vi "Recalibration.vi"() -> ()   [LabVIEW 2012]
uses:
  <vilib>/Utility/file.llb/Read From Spreadsheet File (I64).vi
  <vilib>/Utility/file.llb/Write To Spreadsheet File (DBL).vi
panel:
  in  "stop":bool
  in  "New\nCalibration #":i32=1 min=1 max=100 step=1
  in  "Correct and Save":bool
  in  "Apply Calibration":bool
  out "Calibration Does Not Exist":bool
  in  "Load Button":bool
  out "Suggested Cal #":i32
  in  "Tolerance (°)":dbl=30.0 min=0.0
  out "Bad Min":bool[](array[boolean])
  out "Bad Max":bool[](array[boolean])
  in  "Calibration #":i32=1 min=1 max=100 step=1
  out "Min Deg":dbl[](array[numeric])
  out "Max Deg":dbl[](array[numeric])
  out "Joint Name":string[](array[string])=["Thumb Roll", "Thumb Inner", "Thumb Outer", "Thm-Ind Abd", "Index MCP", "Index PIP", "Middle MCP", "Middle PIP", "Ind-Mid Abd", "Ring MCP", "Ring PIP", "Mid-Rng Abd", "Pinkie MCP", "Pinkie PIP", "Rng-Pnk Abduction", "Wrist Pitch", "Wrist Yaw"]
  out "Min Raw":i64[](array[numeric])
  out "Max Raw":i64[](array[numeric])
  in  "Hand":string(combo)="LH"
  in  "Subject Initials":string="Default"
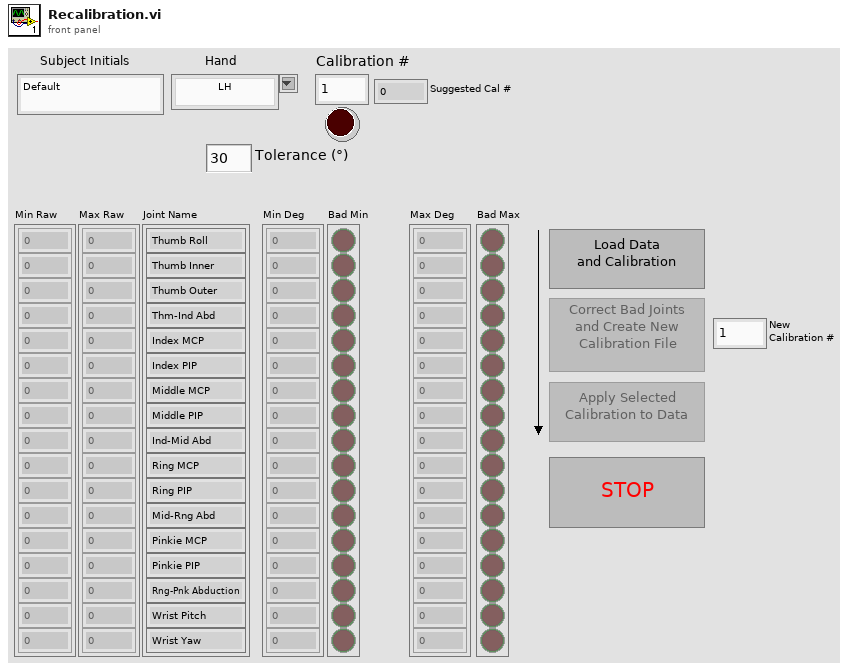
[diagram p1: front panel]
types:
  T1 = enum8{"Enabled", "Disabled", "Disabled and Grayed Out"}
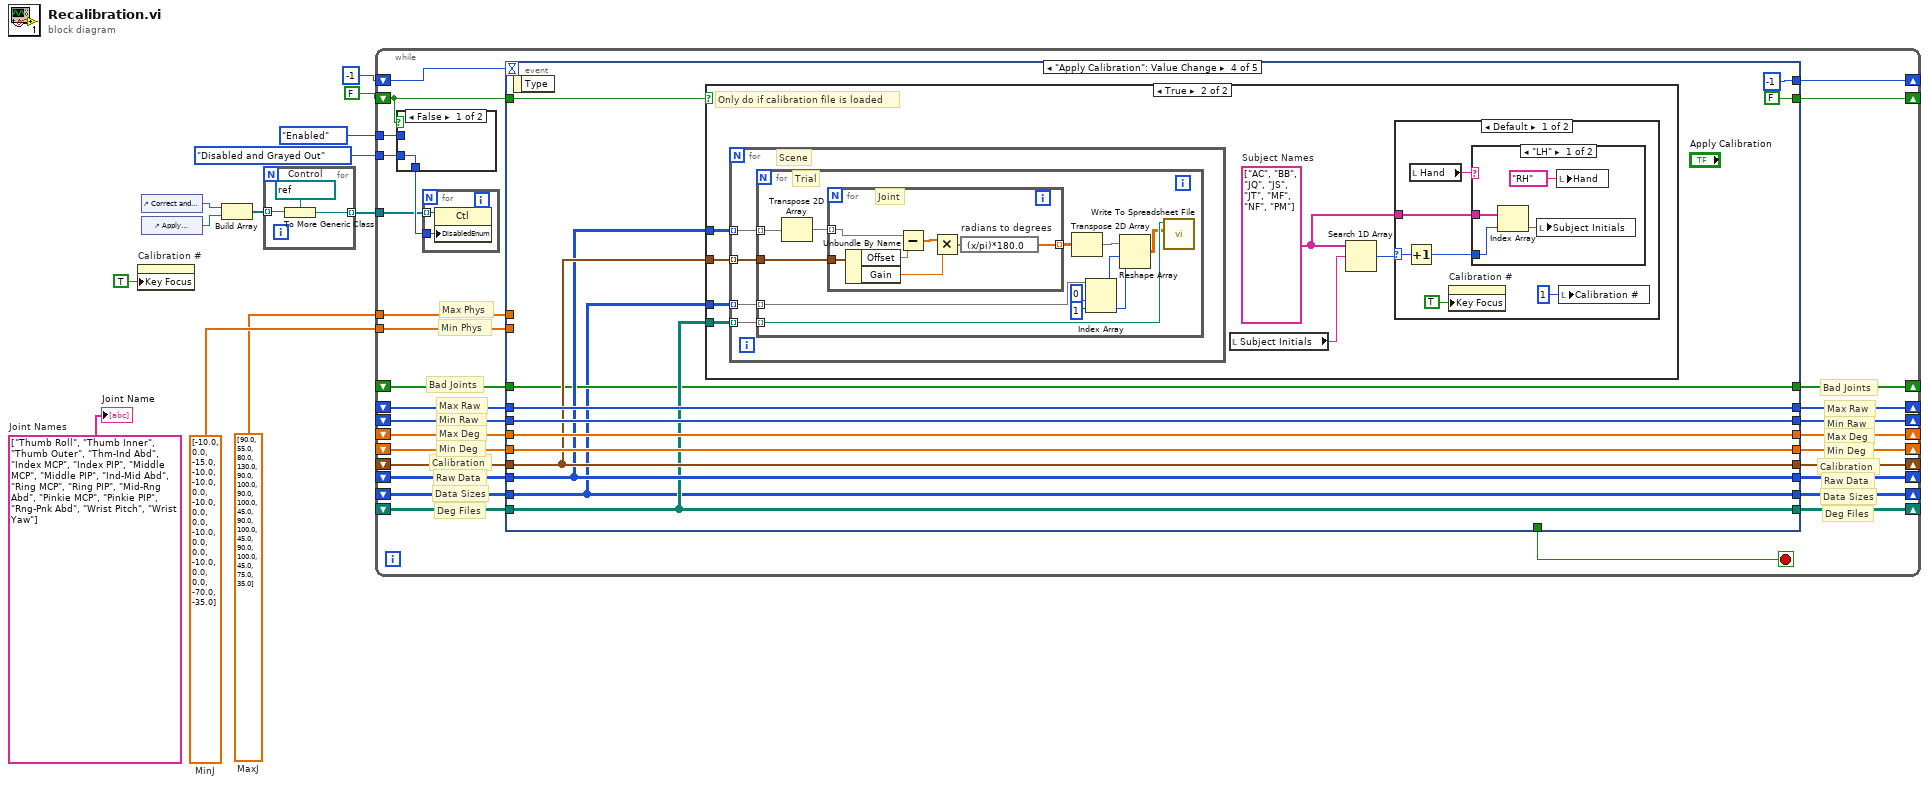
[diagram p0: block diagram]
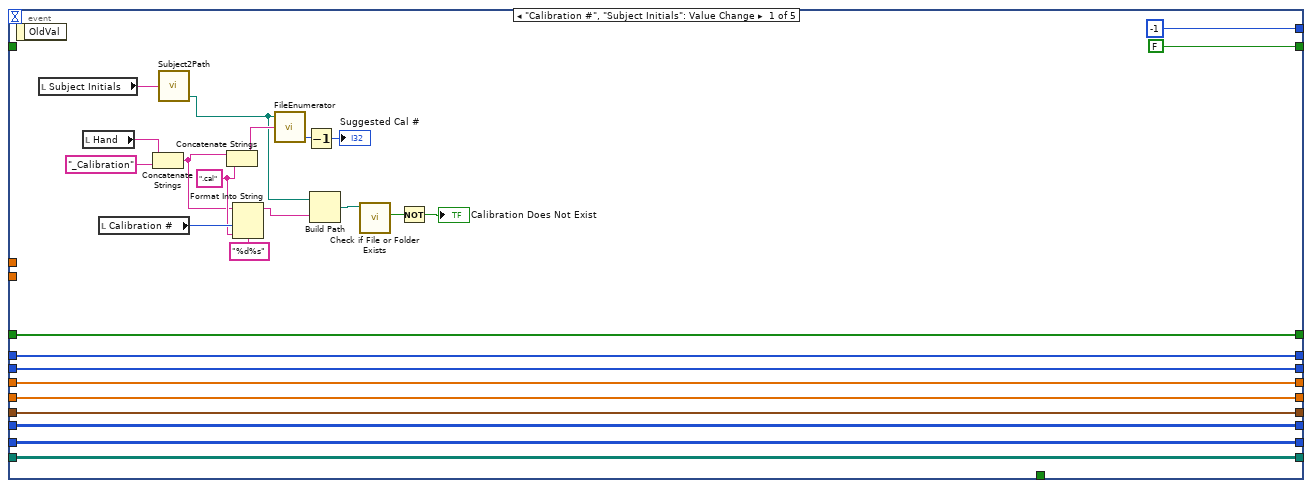
[diagram p3: hidden frame]
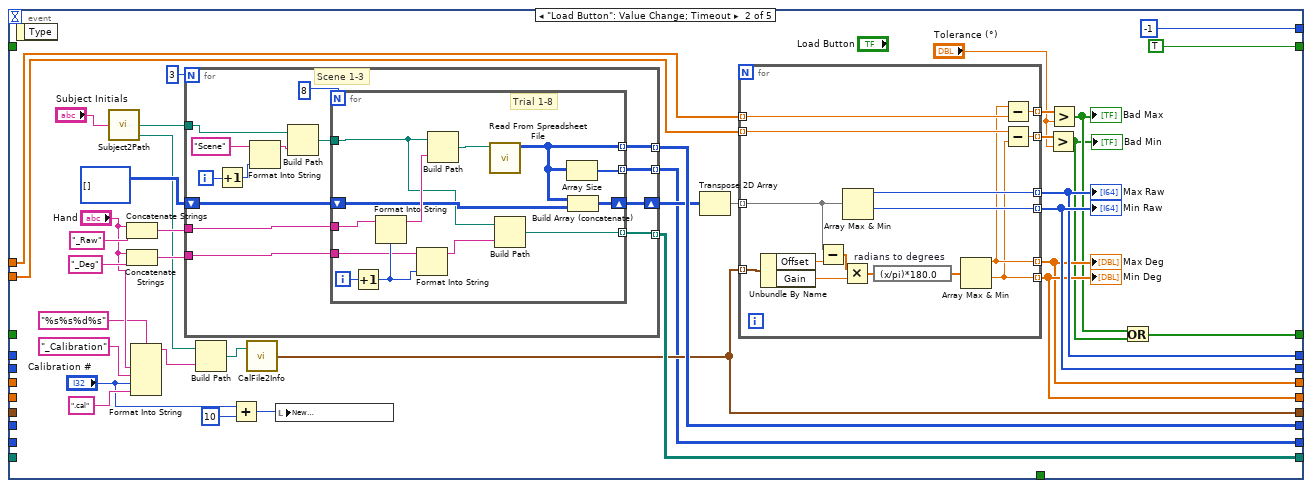
[diagram p4: hidden frame]
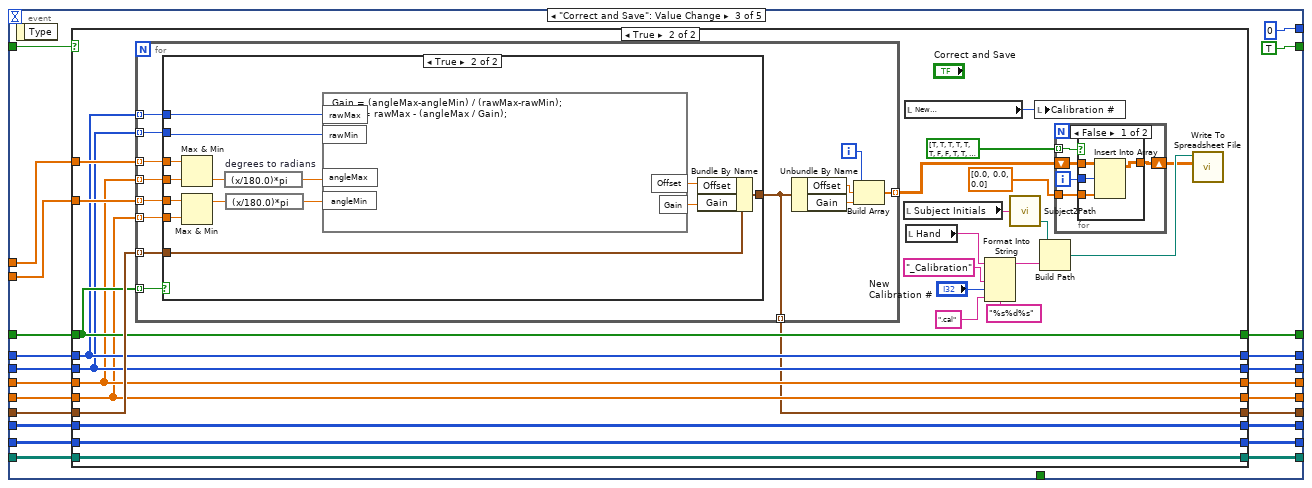
[diagram p5: hidden frame]
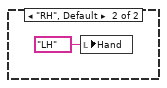
[diagram p10: hidden frame]
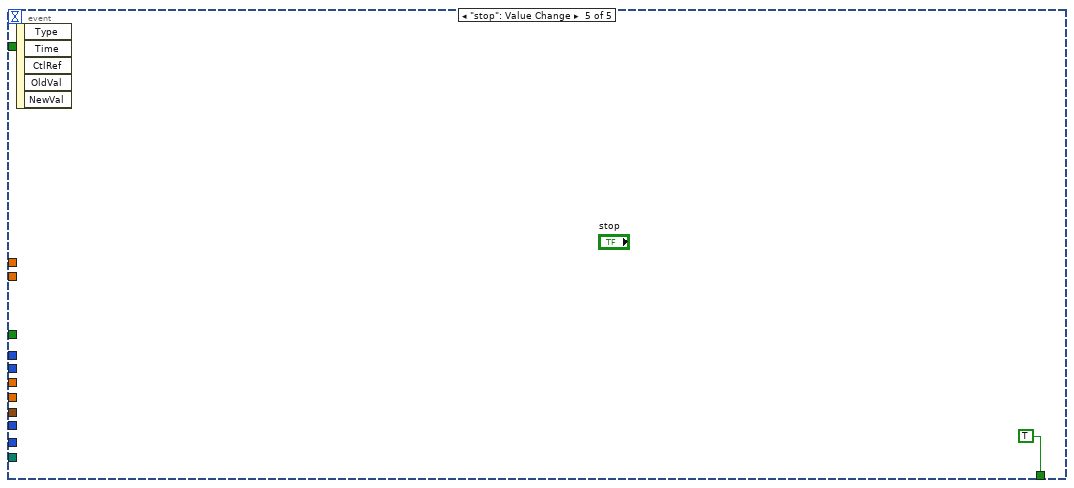
[diagram p12: hidden frame]
diagram:
  w9 = dbl[] [90.0, 55.0, 80.0, 130.0, 90.0, 100.0, 90.0, 100.0, 45.0, 90.0, 100.0, 45.0, 90.0, 100.0, 45.0, 75.0, 35.0]  # MaxJ
  w10 = dbl[] [-10.0, 0.0, -15.0, -10.0, -10.0, 0.0, -10.0, 0.0, 0.0, -10.0, 0.0, 0.0, -10.0, 0.0, 0.0, -70.0, -35.0]  # MinJ
  w11 = string[] ["Thumb Roll", "Thumb Inner", "Thumb Outer", "Thm-Ind Abd", "Index MCP", "Index PIP", "Middle MCP", "Middle PIP", "Ind-Mid Abd", "Ring MCP", "Ring PIP", "Mid-Rng Abd", "Pinkie MCP", "Pinkie PIP", "Rng-Pnk Abd", "Wrist Pitch", "Wrist Yaw"]  # Joint Names
  n1 = property on="Calibration #" class="DigNum (strict)"("Key Focus"=TRUE) -> ()  [unwired: 2 in, 2 out]
  n2 = control-ref of="Correct and Save"() -> (w7:refnum<vi>)
  n3 = control-ref of="Apply Calibration"() -> (w6:refnum<vi>)
  n4 = Build Array(w7, w6) -> (w5:refnum<vi>[])
  n5 = for {
    tunnel: w5 -> [w15] mode=indexing
    tunnel: [w13] -> w2 mode=indexing
    w14 = refnum<vi> refnum  # Control
    n6 = To More Generic Class(target class=w14, reference=w15) -> (generic class reference=w13:refnum<vi>)
  }
  n7 = while {
    shift-right: [w44] -> _
    shift-left: _ -> [w43]
    shift-right: [w42] -> _
    shift-left: _ -> [w31]
    shift-right: [w41] -> _
    shift-left: _ -> [w32]
    shift-right: [w37] -> _
    shift-left: _ -> [w33]
    shift-right: [w38] -> _
    shift-left: _ -> [w34]
    shift-right: [w39] -> _
    shift-left: _ -> [w35]
    shift-right: [w40] -> _
    shift-left: _ -> [w36]
    shift-right: [w30] -> _
    shift-left: FALSE ("Load Button") -> [w20]
    tunnel: w10 -> [w29]
    tunnel: w9 -> [w28]
    shift-right: [w27] -> _
    shift-left: _ -> [w26]
    shift-right: [w25] -> _
    shift-left: -1 -> [w24]
    shift-right: [w22] -> _
    shift-left: _ -> [w21]
    tunnel: T1."Enabled" ("Disabled") -> [w19]
    tunnel: T1."Disabled and Grayed Out" ("Disabled") -> [w18]
    tunnel: w2 -> [w16]
    stop <- w23 stop-if-true
    # "Data Sizes"
    # "Data Sizes"
    # "Bad Joints"
    # "Bad Joints"
    # "Min Phys"
    # "Max Phys"
    # "Deg Files"
    # "Raw Data"
    # "Calibration"
    # "Min Deg"
    # "Max Deg"
    # "Min Raw"
    # "Max Raw"
    # "Deg Files"
    # "Raw Data"
    # "Calibration"
    # "Min Deg"
    # "Max Deg"
    # "Min Raw"
    # "Max Raw"
    n8 = case shown="False" w20 {
      tunnel: w19 -> [_ w48]
      tunnel: w18 -> [w47 _]
      tunnel: [w47 w48] -> w17
      frame False {
      }
      frame True {
      }
    }
    n9 = for {
      tunnel: w17 -> [w46]
      tunnel: w16 -> [w45] mode=indexing
      n10 = property class="Ctl"(reference=w45, "DisabledEnum"=w46) -> ()  [unwired: 1 in, 2 out]
    }
    n11 = event shown="[3] \"Apply Calibration\": Value Change" {
      selector: _ -> [_ _ _ _ _]
      dyn-events: _ -> [_ _ _ _ _]
      timeout: w24 -> [_ _ _ _ _]
      tunnel: [w69 w95 w166 w258 _] -> w44
      tunnel: w43 -> [w69 _ w171 w258 _]
      tunnel: [w63 w98 w169 w256 _] -> w42
      tunnel: [w64 w97 w167 w257 _] -> w41
      tunnel: [w68 w92 w162 w262 _] -> w40
      tunnel: [w67 w93 w163 w261 _] -> w39
      tunnel: [w66 w90 w164 w260 _] -> w38
      tunnel: [w65 w91 w165 w259 _] -> w37
      tunnel: w36 -> [w68 _ w175 w262 _]
      tunnel: w35 -> [w67 _ w174 w261 _]
      tunnel: w34 -> [w66 _ w173 w260 _]
      tunnel: w33 -> [w65 _ w172 w259 _]
      tunnel: w32 -> [w64 _ w170 w257 _]
      tunnel: w31 -> [w63 _ w168 w256 _]
      tunnel: [FALSE ("Load Button") TRUE ("Load Button") TRUE ("Load Button") FALSE ("Load Button") _] -> w30
      tunnel: w20 -> [_ _ w177 w255 _]
      tunnel: w29 -> [_ w87 w159 _ _]
      tunnel: w28 -> [_ w88 w160 _ _]
      tunnel: [w52 w78 w161 w254 _] -> w27
      tunnel: w26 -> [w52 _ w176 w254 _]
      tunnel: [-1 -1 0 -1 _] -> w25
      tunnel: [_ _ _ _ TRUE] -> w23
      tunnel: [w49 w75 w155 w251 _] -> w22
      tunnel: w21 -> [w49 _ w156 w251 _]
      event "Calibration #", "Subject Initials": Value Change {
        w60 = ".cal"
        n12 = event-data() -> ()  [unwired: 1 in, 1 out]
        n13 = local read "Subject Initials"() -> (w74:string)
        n14 = local read "Hand"() -> (w73:string)
        n15 = local read "Calibration #"() -> (w61:i32)
        n16 = Concatenate Strings(w73, "_Calibration") -> (w59:string)
        n17 = call "Subject2Path.vi"("Subject Initials"=w74) -> ("Calibration Path"=w57:path)  [unwired: 1 in, 2 out]
        n18 = Concatenate Strings(w59, w60) -> (w62:string)
        n19 = Format Into String(format string="%d%s", initial string=w59, w61, w60) -> (resulting string=w56:string)  [unwired: 1 in, 1 out]
        n20 = call "FileEnumerator.vi"("Filename"=w62, "Path"=w57) -> ("Number"=w70:i32)  [unwired: 1 in, 2 out]
        n21 = Decrement(x=w70) -> (x-1=→"Suggested Cal #":i32)
        n22 = Build Path(base path=w57, name or relative path=w56) -> (appended path=w55:path)
        n23 = call <vilib>:"Check if File or Folder Exists.vi"("path"=w55) -> ("file or folder exists?"=w54:bool)  [unwired: 8 in, 2 out]
        n24 = Not(x=w54) -> (.not. x?=→"Calibration Does Not Exist":bool)
      }
      event "Load Button": Value Change; Timeout {
        n25 = event-data() -> ()  [unwired: 1 in, 1 out]
        n26 = call "Subject2Path.vi"("Subject Initials"="Subject Initials") -> ("Data Path"=w105:path, "Calibration Path"=w100:path)  [unwired: 1 in, 1 out]
        n27 = Concatenate Strings("Hand", "_Raw") -> (w108:string)
        n28 = Concatenate Strings("Hand", "_Deg") -> (w107:string)
        n29 = Format Into String(format string="%s%s%d%s", "Hand", "_Calibration", "Calibration #", ".cal") -> (resulting string=w99:string)  [unwired: 2 in, 1 out]
        n30 = for {
          N: 3 -> [_]
          tunnel: w105 -> [w138]
          tunnel: w108 -> [w136]
          shift-right: [w132] -> w96
          shift-left: i64[][] [] ("array") -> [w133]
          tunnel: [w131] -> w97 mode=indexing
          tunnel: w107 -> [w130]
          tunnel: [w129] -> w98 mode=indexing
          tunnel: [w128] -> w75 mode=indexing
          i -> [w140]
          # "Scene 1-3"
          n31 = Increment(x=w140) -> (x+1=w139:i32)
          n32 = Format Into String(initial string="Scene", w139) -> (resulting string=w134:string)  [unwired: 2 in, 1 out]
          n33 = Build Path(base path=w138, name or relative path=w134) -> (appended path=w137:path)
          n34 = for {
            N: 8 -> [_]
            tunnel: w137 -> [w146]
            tunnel: w136 -> [w153]
            shift-right: [w149] -> w132
            shift-left: w133 -> [w150]
            tunnel: [w143] -> w131 mode=indexing
            tunnel: w130 -> [w147]
            tunnel: [w144] -> w129 mode=indexing
            tunnel: [w142] -> w128 mode=indexing
            i -> [w154]
            # "Trial 1-8"
            n35 = Increment(x=w154) -> (x+1=w148:i32)
            n36 = Format Into String(initial string=w153, w148) -> (resulting string=w152:string)  [unwired: 2 in, 1 out]
            n37 = Format Into String(initial string=w147, w148) -> (resulting string=w145:string)  [unwired: 2 in, 1 out]
            n38 = Build Path(base path=w146, name or relative path=w152) -> (appended path=w151:path)
            n39 = call-poly <vilib>:"Read From Spreadsheet File.vi"("file path (dialog if empty)"=w151) -> ("all rows"=w143:i64[][])  [unwired: 6 in, 4 out]
            n40 = Build Path(base path=w146, name or relative path=w145) -> (appended path=w144:path)
            n41 = Array Size(array=w143) -> (size(s)=w142:i32[])
            n42 = Build Array (concatenate)(w143, w150) -> (w149:i64[][])
          }
        }
        n43 = Build Path(base path=w100, name or relative path=w99) -> (appended path=w89:path)
        n44 = Add(x="Calibration #", y=10) -> (x+y=w81:i32)
        n45 = call "CalFile2Info.vi"("Calibration File"=w89) -> ("Calibration Array"=w95:cluster{"Offset":dbl, "Gain":dbl}[])  [unwired: 3 in]
        n46 = local write "New\nCalibration #"(w81) -> ()
        n47 = Transpose 2D Array(2D array=w96) -> (transposed array=w94:i64[][])
        n48 = for {
          tunnel: w95 -> [w127] mode=indexing
          tunnel: w94 -> [w121] mode=indexing
          tunnel: [w120] -> w92 mode=indexing
          tunnel: [w119] -> w93 mode=indexing
          tunnel: [w116] -> w90 mode=indexing
          tunnel: [w115] -> w91 mode=indexing
          tunnel: w88 -> [w118] mode=indexing
          tunnel: w87 -> [w117] mode=indexing
          tunnel: [w114] -> w86 mode=indexing
          tunnel: [w113] -> w85 mode=indexing
          n49 = Unbundle By Name(w127) -> ("Offset"=w126:dbl, "Gain"=w125:dbl)
          n50 = Subtract(x=w121, y=w126) -> (x-y=w124:dbl[])
          n51 = Multiply(x=w124, y=w125) -> (x*y=w123:dbl[])
          n52 = Array Max & Min(array=w121) -> (max value=w120:i64, min value=w119:i64)  [unwired: 2 out]
          n53 = expression code="(x/pi)*180.0" "radians to degrees"(w123) -> (w122:dbl[])
          n54 = Array Max & Min(array=w122) -> (max value=w116:dbl, min value=w115:dbl)  [unwired: 2 out]
          n55 = Subtract(x=w116, y=w118) -> (x-y=w114:dbl)
          n56 = Subtract(x=w117, y=w115) -> (x-y=w113:dbl)
        }
        "Min Raw" <- w93
        "Max Raw" <- w92
        "Min Deg" <- w91
        "Max Deg" <- w90
        n57 = Greater?(x=w85, y="Tolerance (°)") -> (0:w79:bool[])
        "Bad Min" <- w79
        n58 = Greater?(x=w86, y="Tolerance (°)") -> (0:w80:bool[])
        "Bad Max" <- w80
        n59 = Or(x=w80, y=w79) -> (x .or. y?=w78:bool[])
      }
      event "Correct and Save": Value Change {
        n60 = event-data() -> ()  [unwired: 1 in, 1 out]
        n61 = case shown="True" w177 {
          tunnel: [w186 w207] -> w161
          tunnel: w176 -> [w186 w207]
          tunnel: [w185 w206] -> w162
          tunnel: w175 -> [w185 w206]
          tunnel: w174 -> [w184 w205]
          tunnel: [w184 w205] -> w163
          tunnel: [w183 w204] -> w164
          tunnel: w173 -> [w183 w204]
          tunnel: [w182 w203] -> w165
          tunnel: w172 -> [w182 w203]
          tunnel: [w181 w202] -> w166
          tunnel: w171 -> [w181 w208]
          tunnel: [w180 w210] -> w167
          tunnel: w170 -> [w180 w210]
          tunnel: [w179 w209] -> w169
          tunnel: w168 -> [w179 w209]
          tunnel: w160 -> [_ w211]
          tunnel: w159 -> [_ w212]
          tunnel: w156 -> [w178 w187]
          tunnel: [w178 w187] -> w155
          frame False {
          }
          frame True {
            n62 = for {
              tunnel: w207 -> [w235] mode=indexing
              tunnel: w206 -> [w234] mode=indexing
              tunnel: w205 -> [w233] mode=indexing
              tunnel: w204 -> [w232] mode=indexing
              tunnel: w203 -> [w231] mode=indexing
              tunnel: w212 -> [w230] mode=indexing
              tunnel: w211 -> [w229] mode=indexing
              tunnel: w208 -> [w228] mode=indexing
              tunnel: [w224] -> w190 mode=indexing
              tunnel: [w223] -> w202 mode=indexing
              i -> [w225]
              n63 = case shown="True" w235 {
                tunnel: w234 -> [_ w250]
                tunnel: w233 -> [_ w249]
                tunnel: w232 -> [_ w246]
                tunnel: w231 -> [_ w245]
                tunnel: w230 -> [_ w244]
                tunnel: w229 -> [_ w243]
                tunnel: w228 -> [w236 w240]
                tunnel: [w236 w237] -> w223
                frame False {
                }
                frame True {
                  n64 = Max & Min(x=w243, y=w246) -> (min(x,y)=w248:dbl)  [unwired: 1 out]
                  n65 = Max & Min(x=w244, y=w245) -> (max(x,y)=w247:dbl)  [unwired: 1 out]
                  n66 = expression code="(x/180.0)*pi" "degrees to radians"(w248) -> (w242:dbl)
                  n67 = expression code="(x/180.0)*pi" ("degrees to radians")(w247) -> (w241:dbl)
                  n68 = formula code="Gain = (angleMax-angleMin) / (rawMax-rawMin);\nOffset = rawMax - (angleMax / Gain);"("angleMax"=w242, "angleMin"=w241, "rawMax"=w250, "rawMin"=w249) -> ("Gain"=w239:dbl, "Offset"=w238:dbl)
                  n69 = Bundle By Name(cluster=w240, "Offset"=w238, "Gain"=w239) -> (w237:cluster{"Offset":dbl, "Gain":dbl})
                }
              }
              n70 = Unbundle By Name(w223) -> ("Offset"=w226:dbl, "Gain"=w227:dbl)
              n71 = Build Array(w225, w226, w227) -> (w224:dbl[])
            }
            n72 = local read "Subject Initials"() -> (w200:string)
            n73 = local read "New\nCalibration #"() -> (w193:i32)
            n74 = local read "Hand"() -> (w197:string)
            n75 = Format Into String(format string="%s%d%s", initial string=w197, "_Calibration", "New\nCalibration #", ".cal") -> (resulting string=w195:string)  [unwired: 1 in, 1 out]
            n76 = call "Subject2Path.vi"("Subject Initials"=w200) -> ("Calibration Path"=w196:path)  [unwired: 1 in, 2 out]
            n77 = local write "Calibration #"(w193) -> ()
            n78 = Build Path(base path=w196, name or relative path=w195) -> (appended path=w194:path)
            n79 = for {
              tunnel: bool[] [TRUE, TRUE, TRUE, TRUE, TRUE, TRUE, FALSE, FALSE, TRUE, TRUE, FALSE, TRUE, TRUE, TRUE, FALSE, TRUE, TRUE, TRUE, FALSE, TRUE, FALSE, TRUE, TRUE, FALSE] ("Sensors Active") -> [w216] mode=indexing
              shift-right: [w215] -> w188
              shift-left: w190 -> [w217]
              tunnel: dbl[] [0.0, 0.0, 0.0] ("new element/subarray") -> [w213]
              i -> [w214]
              n80 = case shown="False" w216 {
                tunnel: w217 -> [w221 w222]
                tunnel: [w220 w222] -> w215
                tunnel: w214 -> [w219 _]
                tunnel: w213 -> [w218 _]
                frame False {
                  n81 = Insert Into Array(array=w221, index (row)=w219, new element=w218) -> (w220:dbl[][])  [unwired: 1 in]
                }
                frame True {
                }
              }
            }
            n82 = call-poly <vilib>:"Write To Spreadsheet File.vi"("2D data"=w188, "file path (dialog if empty)"=w194) -> ()  [unwired: 6 in, 1 out]
          }
        }
      }
      event "Apply Calibration": Value Change {
        n83 = event-data() -> ()  [unwired: 1 in, 1 out]
        n84 = case shown="True" w255 {
          tunnel: w258 -> [_ w269]
          tunnel: w257 -> [_ w268]
          tunnel: w256 -> [_ w267]
          tunnel: w251 -> [_ w266]
          frame False {
          }
          frame True {
            w263 = string[] ["AC", "BB", "JQ", "JS", "JT", "MF", "NF", "PM"]  # Subject Names
            # "Only do if calibration file is loaded"
            n85 = for {
              tunnel: w268 -> [w284] mode=indexing
              tunnel: w269 -> [w283] mode=indexing
              tunnel: w267 -> [w282] mode=indexing
              tunnel: w266 -> [w281] mode=indexing
              # "Scene"
              n86 = for {
                tunnel: w284 -> [w296] mode=indexing
                tunnel: w283 -> [w294]
                tunnel: w282 -> [w292] mode=indexing
                tunnel: w281 -> [w288] mode=indexing
                # "Trial"
                n87 = Transpose 2D Array(2D array=w296) -> (transposed array=w295:i64[][])
                n88 = for {
                  tunnel: w295 -> [w302] mode=indexing
                  tunnel: w294 -> [w303]
                  tunnel: [w297] -> w293 mode=indexing
                  # "Joint"
                  n89 = Unbundle By Name(w303) -> ("Offset"=w301:dbl, "Gain"=w299:dbl)
                  n90 = Subtract(x=w302, y=w301) -> (x-y=w300:dbl[])
                  n91 = Multiply(x=w300, y=w299) -> (x*y=w298:dbl[])
                  n92 = expression code="(x/pi)*180.0" "radians to degrees"(w298) -> (w297:dbl[])
                }
                n93 = Transpose 2D Array(2D array=w293) -> (transposed array=w291:dbl[][])
                n94 = Index Array(array=w288, index #1=0 ("index"), index #2=1 ("index")) -> (element #1=w287:i32, element #2=w286:i32)
                n95 = Reshape Array(w291, w287, w286) -> (w285:dbl[][])
                n96 = call-poly <vilib>:"Write To Spreadsheet File.vi"("2D data"=w285, "file path (dialog if empty)"=w292) -> ()  [unwired: 6 in, 1 out]
              }
            }
            n97 = local read "Subject Initials"() -> (w265:string)
            n98 = Search 1D Array(1D array=w263, element=w265) -> (index of element=w264:i32)  [unwired: 1 in]
            n99 = case shown="Default" w264 {
              selector: w264 -> [w273 _]
              tunnel: w263 -> [w274 _]
              frame Default {
                n100 = Increment(x=w273) -> (x+1=w272:i32)
                n101 = local read "Hand"() -> (w275:string)
                n102 = property on="Calibration #" class="DigNum (strict)"("Key Focus"=TRUE) -> ()  [unwired: 2 in, 2 out]
                n103 = case shown="\"LH\"" w275 {
                  tunnel: w274 -> [w278 _]
                  tunnel: w272 -> [w277 _]
                  frame "LH" {
                    n104 = Index Array(array=w278, index=w277) -> (element=w276:string)
                    n105 = local write "Subject Initials"(w276) -> ()
                    n106 = local write "Hand"("RH" ("Hand")) -> ()
                  }
                  frame "RH", Default {
                    n107 = local write "Hand"("LH" ("Hand")) -> ()
                  }
                }
                n108 = local write "Calibration #"(1 ("Calibration #")) -> ()
              }
              frame -1 {
              }
            }
          }
        }
      }
      event "stop": Value Change {
        n109 = event-data() -> ()  [unwired: 1 in, 5 out]
      }
    }
  }
  "Joint Name" <- w11
